vi "Send set temperature.vi"(8 "error in (no error)":errorcluster, 10 "TEMP":string, 11 "Channel in":refnum<class "Channel.lvclass">) -> (0 "error out":errorcluster, 3 "Channel out":refnum<class "Channel.lvclass">)   [LabVIEW 2018, in "Channel.lvclass"]
uses:
  Channel.lvclass
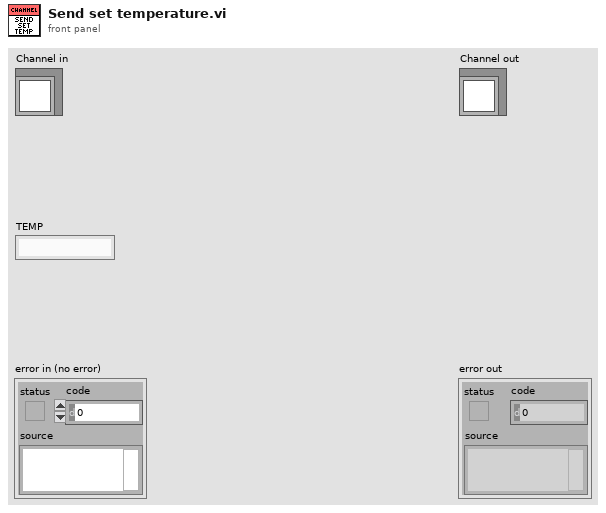
[diagram p1: front panel]
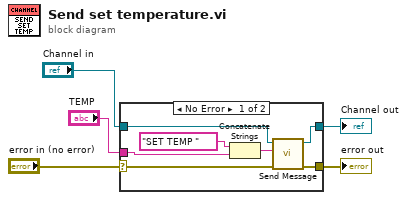
[diagram p0: block diagram]
diagram:
  n1 = case shown="No Error" "error in (no error)" {
    selector: "error in (no error)" -> [w9 w14]
    tunnel: [w12 w14] -> w4
    tunnel: [w11 w13] -> w2
    tunnel: "Channel in" -> [w10 w13]
    tunnel: "TEMP" -> [w6 _]
    frame No Error {
      n2 = Concatenate Strings("SET TEMP ", w6) -> (w7:string)
      n3 = call "Send Message.vi"("error in (no error)"=w9, "message"=w7, "Channel in"=w10) -> ("error out"=w12:errorcluster, "Channel out"=w11:refnum<class "Channel.lvclass">)  [unwired: 7 in]
    }
    frame Error {
    }
  }
  "error out" <- w4
  "Channel out" <- w2
